vi "Send Command.vi"(8 "error in":errorcluster, 9 "Value":variant, 10 "Command":string, 11 "CrossPoint in":refnum<class "CrossPoint.lvclass">) -> (0 "error out":errorcluster, 3 "CrossPoint out":refnum<class "CrossPoint.lvclass">)   [LabVIEW 2019, in "CrossPoint.lvlib" / "CrossPoint.lvclass"]
uses:
  Library/CrossPoint.lvclass
  builds/Instruments/Instruments.lvlibp/Library/Instruments.lvclass
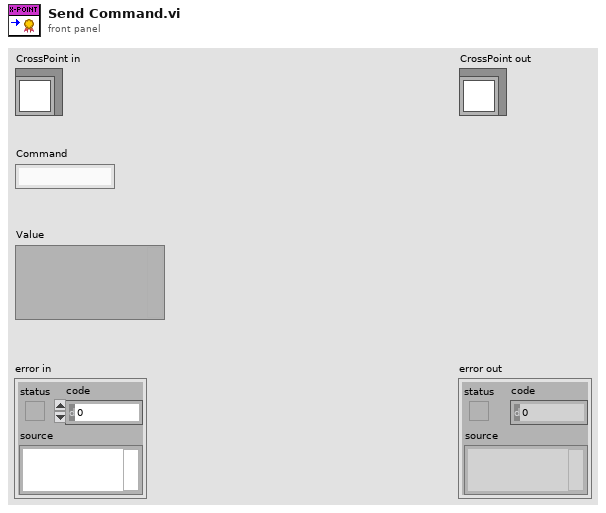
[diagram p1: front panel]
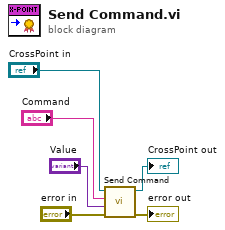
[diagram p0: block diagram]
diagram:
  n1 = call-parent "Send Command.vi"("error in"="error in", "Value"="Value", "Command"="Command", "Instruments in"="CrossPoint in") -> ("error out"=→"error out":errorcluster, "Instruments out"=→"CrossPoint out":refnum<class "CrossPoint.lvclass">)  [unwired: 6 in]
